vi "Report.vi"(8 "error in (no error)":errorcluster, 9 "Received":path, 10 "Approved":path, 11 "LVCompare in":refnum<class "LVCompare.lvclass">) -> (0 "error out":errorcluster, 3 "LVCompare out":refnum<class "LVCompare.lvclass">)   [LabVIEW 2020, in "Approval Tests.lvlib" / "LVCompare.lvclass"]
uses:
  LVCompare.lvclass
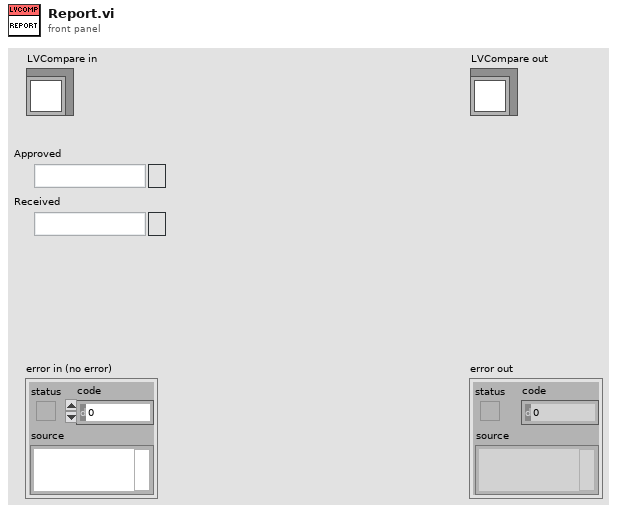
[diagram p1: front panel]
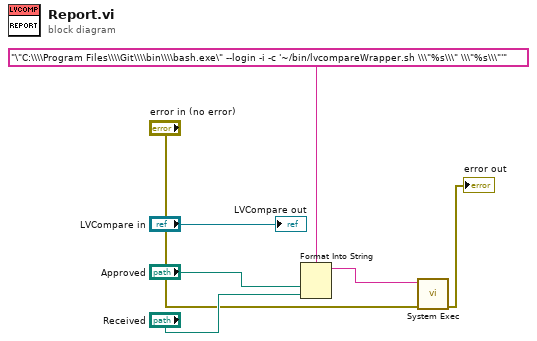
[diagram p0: block diagram]
diagram:
  n1 = Format Into String(format string="\"C:\\\\Program Files\\\\Git\\\\bin\\\\bash.exe\" --login -i -c '~/bin/lvcompareWrapper.sh \\\"%s\\\" \\\"%s\\\"'", "Approved", "Received") -> (resulting string=w3:string)  [unwired: 2 in, 1 out]
  n2 = call <vilib>:"System Exec.vi"("error in (no error)"="error in (no error)", "command line"=w3) -> ("error out"=→"error out":errorcluster)  [unwired: 6 in, 3 out]
  "LVCompare out" <- "LVCompare in"
